vi "Actor Launched.vi"(5 "Actor Type":string, 7 "Actor Cores":string[](array[string]), 8 "error in (no error)":errorcluster, 9 "Actor's Caller Q":refnum<class "Message Enqueuer.lvclass">, 10 "Actor's Self Q":refnum<class "Message Enqueuer.lvclass">, 11 "Monitor Data in":refnum<class "Monitor Data.lvclass">) -> (0 "error out":errorcluster, 3 "Monitor Data out":refnum<class "Monitor Data.lvclass">)   [LabVIEW 2017, in "MGI-Monitored Actor Core.lvlib" / "Monitor Data.lvclass"]
doc: "Add the new actor to the data store\n\nCopyright: MGI 2016\nAuthor: Derek Trepanier"
uses:
  Monitor Data.lvclass
  <vilib>/ActorFramework/Message Enqueuer/Message Enqueuer.lvclass
  Monitor Data.lvclass/Monitor Data.ctl
  Actor Data.ctl
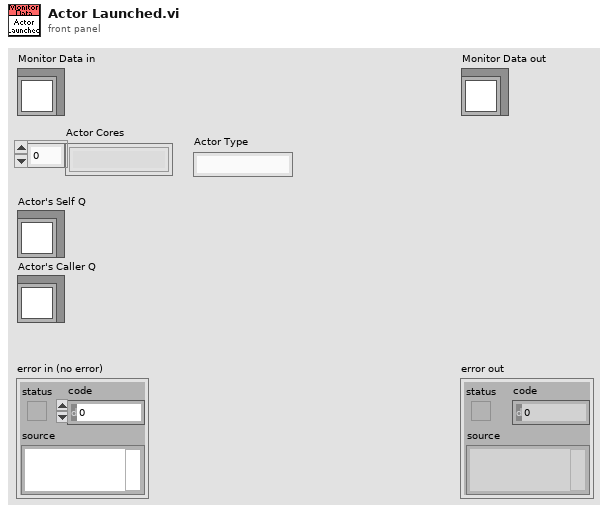
[diagram p1: front panel]
types:
  T1 = typedef "MGI-Monitored Actor Core.lvlib/Monitor Data.lvclass/Actor Data.ctl" = cluster{"Actor Type":string, "Actor Cores":string[], "Self":refnum<class "Message Enqueuer.lvclass">, "Caller":refnum<class "Message Enqueuer.lvclass">, "Actor Label":string, "Last Ping":dbl}
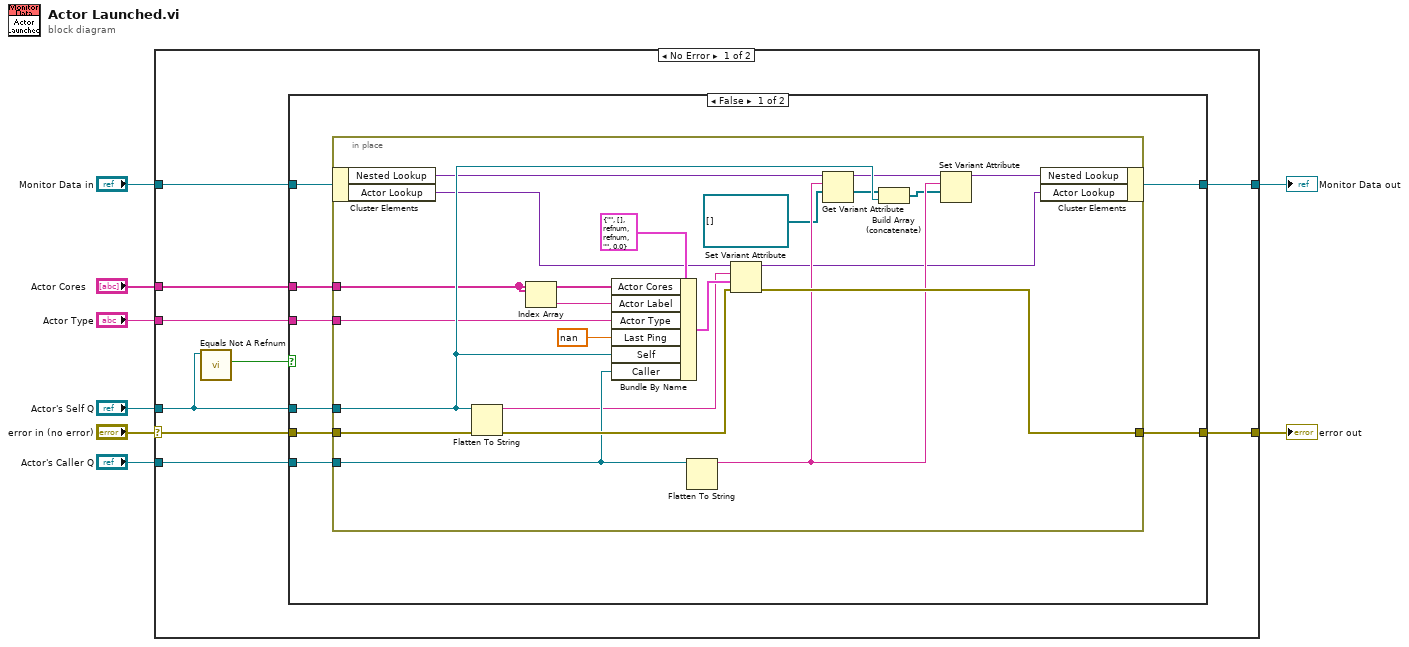
[diagram p0: block diagram]
diagram:
  n1 = case shown="No Error" "error in (no error)" {
    selector: "error in (no error)" -> [w12 w50]
    tunnel: [w13 w50] -> w6
    tunnel: [w14 w49] -> w7
    tunnel: "Monitor Data in" -> [w15 w49]
    tunnel: "Actor's Self Q" -> [w10 _]
    tunnel: "Actor Cores" -> [w17 _]
    tunnel: "Actor's Caller Q" -> [w16 _]
    tunnel: "Actor Type" -> [w11 _]
    frame No Error {
      n2 = call <vilib>:"Equals Not A Refnum.vi"("Message Enqueuer"=w10) -> ("Not a refnum?"=w9:bool)  [unwired: 10 in]
      n3 = case shown="False" w9 {
        tunnel: w10 -> [w25 _]
        tunnel: w17 -> [w24 _]
        tunnel: w16 -> [w23 _]
        tunnel: w15 -> [w22 w48]
        tunnel: [w21 w48] -> w14
        tunnel: [w20 w47] -> w13
        tunnel: w12 -> [w19 w47]
        tunnel: w11 -> [w18 _]
        frame False {
          n4 = in-place {
            in-place-border: w25 -> [w41]
            in-place-border: [w44] -> w20
            in-place-border: w24 -> [w27]
            in-place-border: w23 -> [w43]
            in-place-border: w19 -> [w31]
            in-place-border: w18 -> [w29]
            n5 = in-place-cluster #1(w22) -> ("Nested Lookup"=w33:variant, "Actor Lookup"=w35:variant)
            n6 = Flatten To String(anything=w41, error in (no error)=w31) -> (data string=w28:string, error out=w46:errorcluster)  [unwired: 2 in, 1 out]
            n7 = Index Array(array=w27) -> (element=w26:string)  [unwired: 1 in]
            n8 = Bundle By Name(cluster=T1 {"Actor Type"="", "Actor Cores"=[], "Self"=refnum, "Caller"=refnum, "Actor Label"="", "Last Ping"=0.0} ("Actor Data"), "Actor Cores"=w27, "Actor Label"=w26, "Actor Type"=w29, "Last Ping"=nan, "Self"=w41, "Caller"=w43) -> (w45:T1)
            n9 = Flatten To String(anything=w43) -> (data string=w40:string)  [unwired: 3 in, 2 out]
            n10 = Set Variant Attribute(Variant=w35, name=w28, value=w45, error in=w46) -> (Variant out=w34:variant, error out=w44:errorcluster)  [unwired: 1 out]
            n11 = Get Variant Attribute(Variant=w33, name=w40, default value (empty Variant)=refnum<class "Message Enqueuer.lvclass">[] []) -> (duplicate Variant=w37:variant, value=w38:refnum<class "Message Enqueuer.lvclass">[])  [unwired: 1 in, 2 out]
            n12 = Build Array (concatenate)(w38, w41) -> (w36:refnum<class "Message Enqueuer.lvclass">[])
            n13 = Set Variant Attribute(Variant=w37, name=w40, value=w36) -> (Variant out=w32:variant)  [unwired: 1 in, 2 out]
            n14 = in-place-cluster #1("Nested Lookup"=w32, "Actor Lookup"=w34) -> (w21:refnum<class "Monitor Data.lvclass">)
          }
        }
        frame True {
        }
      }
    }
    frame Error {
    }
  }
  "error out" <- w6
  "Monitor Data out" <- w7
